vi "Close Connection.vi"(8 "error in (no error)":errorcluster, 11 "object in":refnum<class "Arduino.lvclass">) -> (0 "error out":errorcluster, 3 "object out":refnum<class "Arduino.lvclass">)   [LabVIEW 2020, in "Arduino.lvclass"]
uses:
  Arduino.lvclass
  Arduino.lvclass/Arduino.ctl
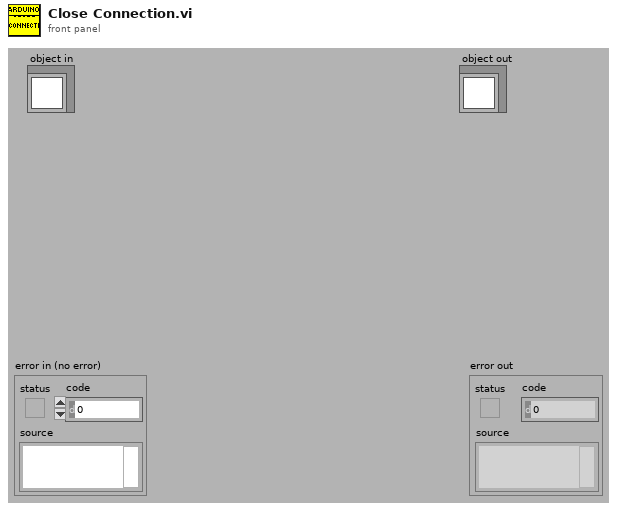
[diagram p1: front panel]
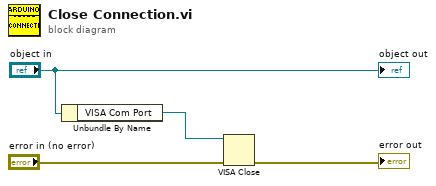
[diagram p0: block diagram]
diagram:
  n1 = Unbundle By Name("object in") -> ("VISA Com Port"=w1:refnum<visa-resource-name>)
  n2 = VISA Close(VISA resource name=w1, error in (no error)="error in (no error)") -> (error out=→"error out":errorcluster)
  "object out" <- "object in"
